vi "Diff Message.vi"(5 "message old":T1, 7 "message new":T1, 10 "change type":T6, 11 "refresh items in":T7[](array[typedef])) -> (3 "refresh items out":T7[](array[typedef]))   [LabVIEW 2020, in "AIM MIL-STD-1553 System Explorer.lvlib" / "Implementation.lvlib" / "Refresh.lvlib"]
uses:
  Refresh.lvlib
  Scripting/Constants.vi
  Scripting/AIM MIL-STD-1553 Scripting.lvlib
  Change Type.ctl
  Shared/Parameter Definition.ctl
  Symbols.ctl
  MCL Row.ctl
  Shared/Address.ctl
  Shared/Terminal Endpoint.ctl
  Shared/Message Type.ctl
  Shared/Message Definition.ctl
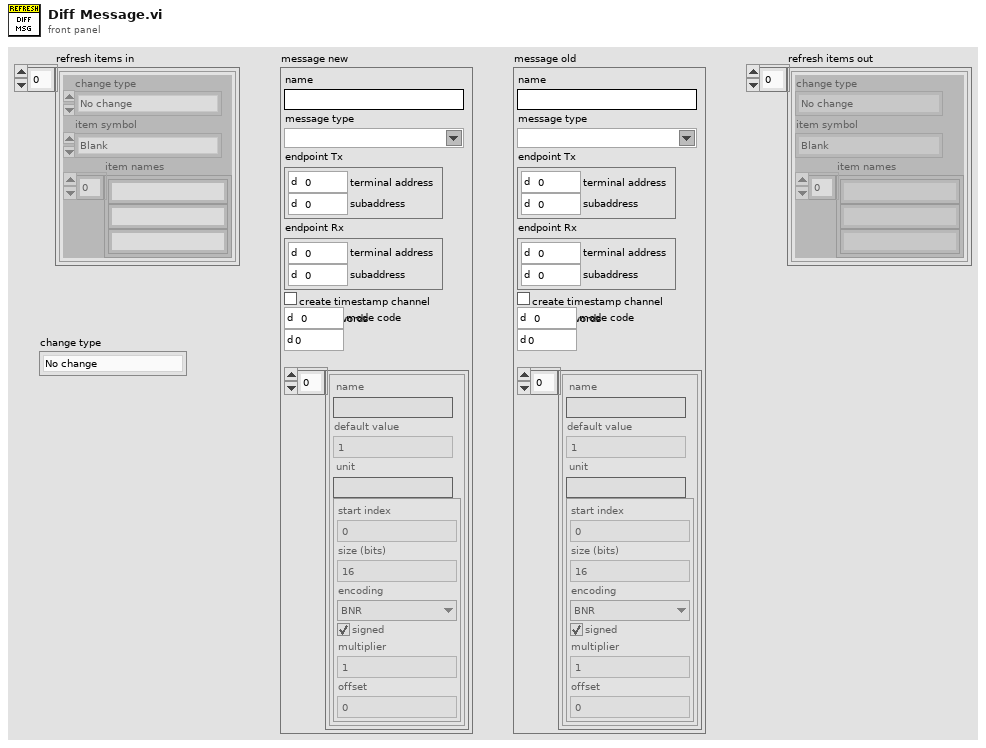
[diagram p1: front panel]
types:
  T1 = typedef "Message Definition.ctl" = cluster{"name":string, "message type":T2, "endpoint Tx":T3, "endpoint Rx":T3, "create timestamp channel":bool, "mode code":u16, "number of words":u16, "parameters":cluster{"name":string, "default value":dbl, "unit":string, "parameter definition":T5}[]}
  T2 = typedef "Message Type.ctl" = string
  T3 = typedef "Terminal Endpoint.ctl" = cluster{"terminal address":T4, "subaddress":T4}
  T4 = typedef "Address.ctl" = u16
  T5 = typedef "Parameter Definition.ctl" = cluster{"start index":i32, "size (bits)":i32, "encoding":enum16{"BNR", "BCD", "Discrete"}, "signed":bool, "multiplier":dbl, "offset":dbl}
  T6 = typedef "AIM MIL-STD-1553 System Explorer.lvlib/Implementation.lvlib/Refresh.lvlib/Change Type.ctl" = enum16{"No change", "Modify", "Add", "Remove"}
  T7 = typedef "AIM MIL-STD-1553 System Explorer.lvlib/Implementation.lvlib/Refresh.lvlib/MCL Row.ctl" = cluster{"change type":T6, "item symbol":T8, "item names":string[]}
  T8 = typedef "AIM MIL-STD-1553 System Explorer.lvlib/Implementation.lvlib/Refresh.lvlib/Symbols.ctl" = enum16{"Blank", "MIL-STD-1553", "Port", "Remote Terminal", "Subaddress", "Bus Controller", "Acyclic Frame", "Mode Code", "Message", "Parameter", "Item"}
  T9 = cluster{"name":string, "default value":dbl, "unit":string, "parameter definition":T5}[]
  T10 = cluster{"name":string, "default value":dbl, "unit":string, "parameter definition":T5}
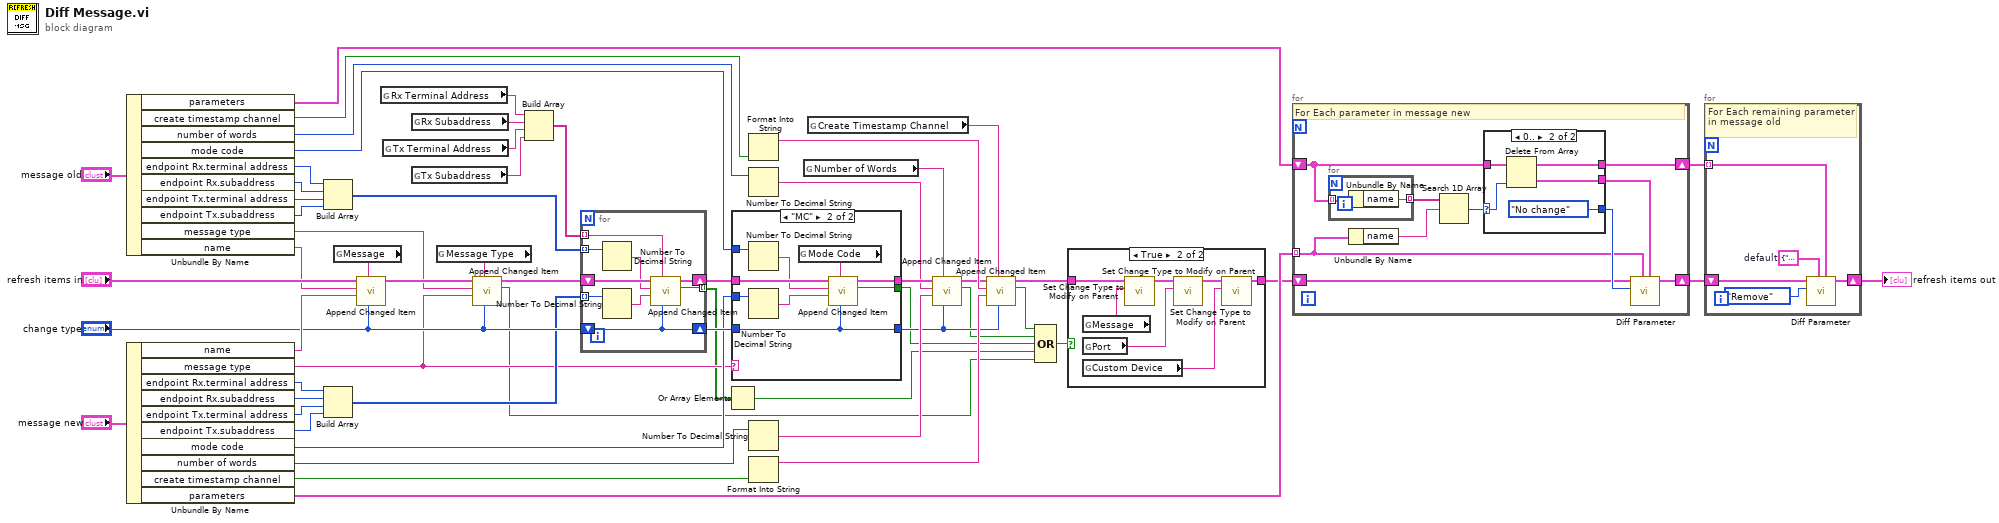
[diagram p0: block diagram]
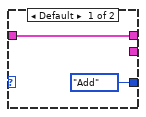
[diagram p2: hidden frame]
diagram:
  n1 = Unbundle By Name("message old") -> ("parameters"=w7:T9, "create timestamp channel"=w1:bool, "number of words"=w2:u16, "mode code"=w30:u16, "endpoint Rx.terminal address"=w47:T4, "endpoint Rx.subaddress"=w46:T4, "endpoint Tx.terminal address"=w45:T4, "endpoint Tx.subaddress"=w44:T4, "message type"=w50:T2, "name"=w54:string)
  n2 = Unbundle By Name("message new") -> ("name"=w53:string, "message type"=w18:T2, "endpoint Rx.terminal address"=w43:T4, "endpoint Rx.subaddress"=w42:T4, "endpoint Tx.terminal address"=w41:T4, "endpoint Tx.subaddress"=w40:T4, "mode code"=w29:u16, "number of words"=w3:u16, "create timestamp channel"=w23:bool, "parameters"=w6:T9)
  n3 = Build Array(w47, w46, w45, w44) -> (w33:T4[])
  n4 = Build Array(w43, w42, w41, w40) -> (w34:T4[])
  n5 = global read "Constants.vi" "Message"() -> (w55:string)
  n6 = call "Append Changed Item.vi"("change type"="change type", "item name"=w55, "new value"=w53, "old value"=w54, "refresh items in"="refresh items in") -> ("refresh items out"=w51:T7[])  [unwired: 5 in, 1 out]
  n7 = global read "Constants.vi" "Rx Terminal Address"() -> (w39:string)
  n8 = global read "Constants.vi" "Tx Terminal Address"() -> (w37:string)
  n9 = global read "Constants.vi" "Rx Subaddress"() -> (w38:string)
  n10 = global read "Constants.vi" "Tx Subaddress"() -> (w36:string)
  n11 = global read "Constants.vi" "Message Type"() -> (w52:string)
  n12 = call "Append Changed Item.vi"("change type"="change type", "item name"=w52, "new value"=w18, "old value"=w50, "refresh items in"=w51) -> ("modify parent"=w13:bool, "refresh items out"=w49:T7[])  [unwired: 5 in]
  n13 = Build Array(w39, w38, w37, w36) -> (w35:string[])
  n14 = for {
    shift-right: [w66] -> w31
    shift-left: w49 -> [w67]
    tunnel: w35 -> [w65] mode=indexing
    tunnel: w34 -> [w64] mode=indexing
    tunnel: w33 -> [w63] mode=indexing
    shift-right: [w60] -> w32
    shift-left: "change type" -> [w60]
    tunnel: [w59] -> w17 mode=indexing
    n15 = Number To Decimal String(number=w63) -> (decimal integer string=w62:string)  [unwired: 1 in]
    n16 = Number To Decimal String(number=w64) -> (decimal integer string=w61:string)  [unwired: 1 in]
    n17 = call "Append Changed Item.vi"("change type"=w60, "item name"=w65, "new value"=w61, "old value"=w62, "refresh items in"=w67) -> ("modify parent"=w59:bool, "refresh items out"=w66:T7[])  [unwired: 5 in]
  }
  n18 = Or Array Elements(Boolean array=w17) -> (logical OR=w10:bool)
  n19 = case shown="\"MC\"" w18 {
    tunnel: w32 -> [w68 w71]
    tunnel: w31 -> [w69 w77]
    tunnel: w30 -> [_ w76]
    tunnel: w29 -> [_ w75]
    tunnel: [w69 w72] -> w27
    tunnel: [w68 w71] -> w19
    tunnel: [_ w70] -> w16
    frame Default {
    }
    frame "MC" {
      n20 = Number To Decimal String(number=w76) -> (decimal integer string=w74:string)  [unwired: 1 in]
      n21 = Number To Decimal String(number=w75) -> (decimal integer string=w73:string)  [unwired: 1 in]
      n22 = global read "Constants.vi" "Mode Code"() -> (w78:string)
      n23 = call "Append Changed Item.vi"("change type"=w71, "item name"=w78, "new value"=w73, "old value"=w74, "refresh items in"=w77) -> ("modify parent"=w70:bool, "refresh items out"=w72:T7[])  [unwired: 5 in]
    }
  }
  n24 = Format Into String(w1) -> (resulting string=w22:string)  [unwired: 3 in, 1 out]
  n25 = Number To Decimal String(number=w2) -> (decimal integer string=w26:string)  [unwired: 1 in]
  n26 = Number To Decimal String(number=w3) -> (decimal integer string=w24:string)  [unwired: 1 in]
  n27 = Format Into String(w23) -> (resulting string=w20:string)  [unwired: 3 in, 1 out]
  n28 = global read "Constants.vi" "Number of Words"() -> (w28:string)
  n29 = global read "Constants.vi" "Create Timestamp Channel"() -> (w25:string)
  n30 = call "Append Changed Item.vi"("change type"=w19, "item name"=w28, "new value"=w24, "old value"=w26, "refresh items in"=w27) -> ("modify parent"=w15:bool, "refresh items out"=w21:T7[])  [unwired: 5 in]
  n31 = call "Append Changed Item.vi"("change type"=w19, "item name"=w25, "new value"=w20, "old value"=w22, "refresh items in"=w21) -> ("modify parent"=w14:bool, "refresh items out"=w11:T7[])  [unwired: 5 in]
  n32 = Compound Arithmetic op=OR(w14, w15, w16, w10, w13) -> (w12:bool)
  n33 = case shown="True" w12 {
    tunnel: w11 -> [w79 w86]
    tunnel: [w79 w83] -> w5
    frame False {
    }
    frame True {
      n34 = global read "Constants.vi" "Message"() -> (w85:string)
      n35 = global read "Constants.vi" "Port"() -> (w81:string)
      n36 = global read "Constants.vi" "Custom Device"() -> (w80:string)
      n37 = call "Set Change Type to Modify on Parent.vi"("parent name"=w85, "refresh items in"=w86) -> ("refresh items out"=w84:T7[])  [unwired: 9 in]
      n38 = call "Set Change Type to Modify on Parent.vi"("parent name"=w81, "refresh items in"=w84) -> ("refresh items out"=w82:T7[])  [unwired: 9 in]
      n39 = call "Set Change Type to Modify on Parent.vi"("parent name"=w80, "refresh items in"=w82) -> ("refresh items out"=w83:T7[])  [unwired: 9 in]
    }
  }
  n40 = for {
    tunnel: w6 -> [w87] mode=indexing
    shift-right: [w93] -> w9
    shift-left: w7 -> [w94]
    shift-right: [w90] -> w8
    shift-left: w5 -> [w88]
    # "For Each parameter in message new"
    n41 = for {
      tunnel: w94 -> [w105] mode=indexing
      tunnel: [w104] -> w95 mode=indexing
      n42 = Unbundle By Name(w105) -> ("name"=w104:string)
    }
    n43 = Unbundle By Name(w87) -> ("name"=w92:string)
    n44 = Search 1D Array(1D array=w95, element=w92) -> (index of element=w96:i32)  [unwired: 1 in]
    n45 = case shown="0.." w96 {
      selector: w96 -> [_ w101]
      tunnel: w94 -> [w98 w103]
      tunnel: [w98 w102] -> w93
      tunnel: [_ w100] -> w89
      tunnel: [Change_Type."Add" ("change type") Change_Type."No change" ("change type")] -> w91
      frame Default {
      }
      frame 0.. {
        n46 = Delete From Array(array=w103, index=w101) -> (deleted portion=w100:T10, array with subset deleted=w102:T9)  [unwired: 1 in]
      }
    }
    n47 = call "Diff Parameter.vi"("parameter old"=w89, "parameter new"=w87, "change type"=w91, "refresh items in"=w88) -> ("refresh items out"=w90:T7[])  [unwired: 7 in]
  }
  n48 = for {
    shift-right: [w110] -> w4
    shift-left: w8 -> [w109]
    tunnel: w9 -> [w107] mode=indexing
    w106 = T10 {"name"="", "default value"=0.0, "unit"="", "parameter definition"={"start index"=0, "size (bits)"=0, "encoding"=enum."BNR", "signed"=FALSE, "multiplier"=0.0, "offset"=0.0}}  # default
    # "For Each remaining parameter in message old"
    n49 = call "Diff Parameter.vi"("parameter old"=w107, "parameter new"=w106, "change type"=Change_Type."Remove", "refresh items in"=w109) -> ("refresh items out"=w110:T7[])  [unwired: 7 in]
  }
  "refresh items out" <- w4
